vi "Close IMU Connection.vi"(8 "Error In":errorcluster, 10 "queue":refnum<queue>, 11 "VISA resource name":refnum<visa-resource-name>) -> (0 "error out":errorcluster)   [LabVIEW 2012]
uses:
  IMU/LabVIEW Library v2/AHRS/SubVI/3DM-GX3-45 Commands/Stop Stream.vi
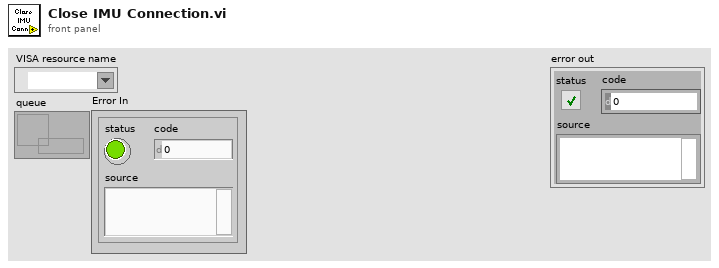
[diagram p1: front panel]
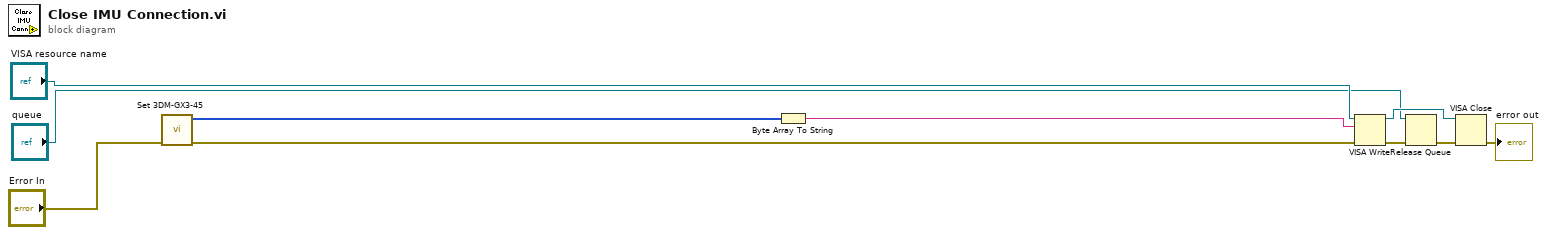
[diagram p0: block diagram]
diagram:
  n1 = call-poly "Set 3DM-GX3-45.vi"("Error In"="Error In") -> ("Error Out"=w8:errorcluster, "Command"=w7:u8[])  [unwired: 9 in]
  n2 = Byte Array To String(unsigned byte array=w7) -> (string=w9:string)
  n3 = VISA Write(VISA resource name="VISA resource name", write buffer=w9, error in (no error)=w8) -> (VISA resource name out=w5:refnum<visa-resource-name>, error out=w6:errorcluster)  [unwired: 1 out]
  n4 = Release Queue(queue="queue", error in (no error)=w6) -> (error out=w10:errorcluster)  [unwired: 1 in, 2 out]
  n5 = VISA Close(VISA resource name=w5, error in (no error)=w10) -> (error out=→"error out":errorcluster)
